vi "WS1050 Calibration.vi"(8 "error in":errorcluster, 9 "OFFSET":bool, 10 "CAPDAC":bool, 11 "I2C Init":bool) -> (0 "error out":errorcluster)   [LabVIEW 2012]
panel:
  in  "Init Data":u8[](array[numeric])=[164, 160, 14, 33] caption="Data Out" format="0x%02x"
  in  "Init Reg":u8[](array[numeric])=[191, 7, 9, 10] caption="Register" format="0x%02x"
  in  "Write Reg I2C":u8=11 caption="Register" format="0x%02x"
  in  "Site Select":T1(ring)
  in  "stop":bool
  in  "READ AD7747":bool
  out "AD7747 Values":string[][](table)
  out "Activity Log":string
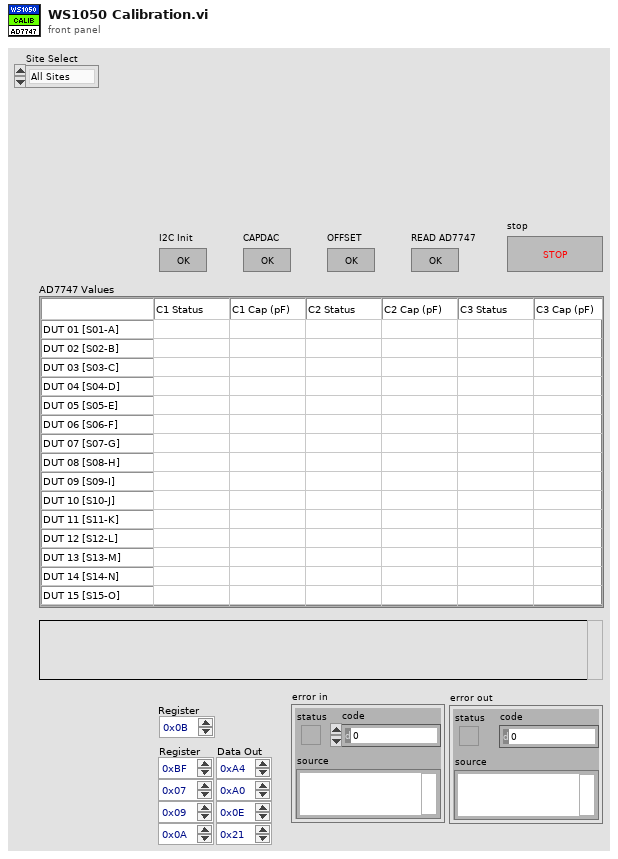
[diagram p1: front panel]
types:
  T1 = enum16{"All Sites", "Site 1", "Site 2", "Site 3"}
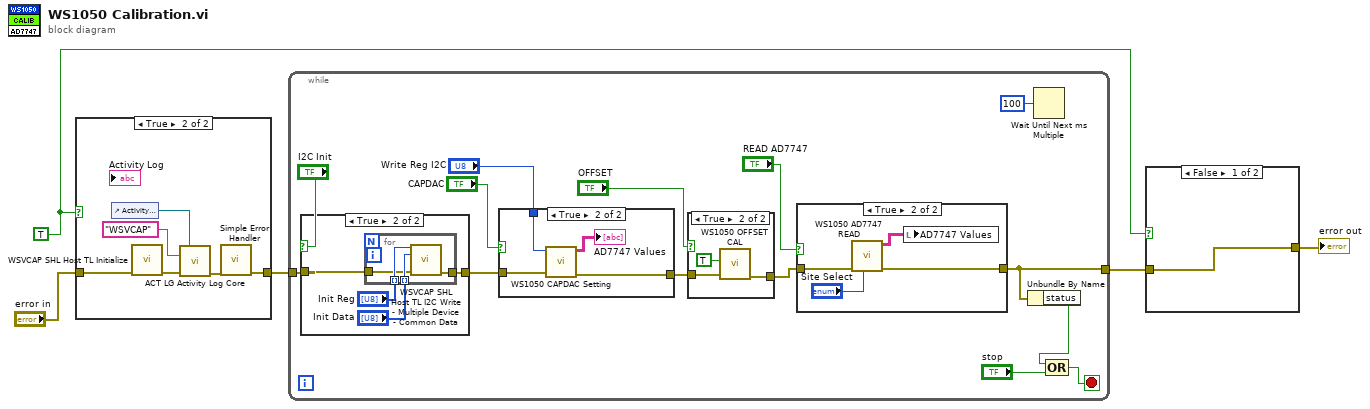
[diagram p0: block diagram]
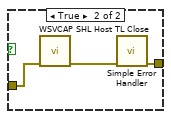
[diagram p6: hidden frame]
diagram:
  w1 = TRUE
  n1 = case shown="True" w1 {
    tunnel: "error in" -> [w6 w8]
    tunnel: [w6 w7] -> w4
    frame False {
    }
    frame True {
      n2 = control-ref of="Activity Log"() -> (w10:refnum<vi>)
      n3 = call "WSVCAP SHL Host TL Initialize.vi"("error in"=w8) -> ("error out"=w12:errorcluster)  [unwired: 14 in]
      n4 = call "ACT LG Activity Log Core.vi"("Display Ref"=w10, "Source"="WSVCAP", "Error In (no error)"=w12) -> ("Error Out"=w11:errorcluster)  [unwired: 11 in, 1 out]
      n5 = call <vilib>:"Simple Error Handler.vi"("error in (no error)"=w11) -> ("error out"=w7:errorcluster)  [unwired: 4 in, 4 out]
    }
  }
  n6 = while {
    tunnel: w4 -> [w14]
    tunnel: [w18] -> w2
    stop <- w19 stop-if-true
    n7 = case shown="True" "I2C Init" {
      tunnel: w14 -> [w27 w31]
      tunnel: [w27 w30] -> w13
      frame False {
      }
      frame True {
        n8 = for {
          tunnel: "Init Reg" -> [w35] mode=indexing
          tunnel: "Init Data" -> [w34] mode=indexing
          tunnel: w31 -> [w33]
          tunnel: [w32] -> w30
          n9 = call "WSVCAP SHL Host TL I2C Write - Multiple Device - Common Data.vi"("Sub Address"=w35, "Data Out [U8]"=w34, "error in"=w33) -> ("error out"=w32:errorcluster)  [unwired: 12 in]
        }
      }
    }
    n10 = case shown="True" "CAPDAC" {
      tunnel: w13 -> [w45 w49]
      tunnel: [w45 w48] -> w26
      tunnel: "Write Reg I2C" -> [_ w46]
      frame False {
      }
      frame True {
        n11 = call "WS1050 CAPDAC Setting.vi"("error in"=w49, "Write Reg I2C"=w46) -> ("error out"=w48:errorcluster, "AD7747 Values"=→"AD7747 Values":string[][])  [unwired: 8 in]
      }
    }
    n12 = case shown="True" "OFFSET" {
      tunnel: w26 -> [w41 w44]
      tunnel: [w41 w43] -> w21
      frame False {
      }
      frame True {
        n13 = call "WS1050 OFFSET CAL.vi"("error in"=w44, "OFFSET CAL"=TRUE) -> ("error out"=w43:errorcluster)  [unwired: 8 in, 1 out]
      }
    }
    n14 = case shown="True" "READ AD7747" {
      tunnel: w21 -> [w36 w40]
      tunnel: [w36 w39] -> w18
      frame False {
      }
      frame True {
        n15 = call "WS1050 AD7747 READ.vi"("Site Select"="Site Select", "error in"=w40) -> ("error out"=w39:errorcluster, "AD7747 Values"=w38:string[][])  [unwired: 8 in]
        n16 = local write "AD7747 Values"(w38) -> ()
      }
    }
    n17 = Unbundle By Name(w18) -> ("status"=w20:bool)
    n18 = Wait Until Next ms Multiple(millisecond multiple=u32 100) -> ()  [unwired: 1 out]
    n19 = Compound Arithmetic op=OR(w20, "stop") -> (w19:bool)
  }
  n20 = case shown="False" w1 {
    tunnel: [w50 w52] -> w3
    tunnel: w2 -> [w50 w51]
    frame False {
    }
    frame True {
      n21 = call "WSVCAP SHL Host TL Close.vi"("error in"=w51) -> ("error out"=w53:errorcluster)  [unwired: 14 in]
      n22 = call <vilib>:"Simple Error Handler.vi"("error in (no error)"=w53) -> ("error out"=w52:errorcluster)  [unwired: 4 in, 4 out]
    }
  }
  "error out" <- w3
